vi "Correction SPOT Open.vi"(8 "error in (no error)":errorcluster, 11 "VISA resource name":refnum<visa-resource-name>) -> (0 "error out":errorcluster, 3 "VISA resource name out":refnum<visa-resource-name>)   [LabVIEW 2014, in "LCR Meter.lvlib"]
doc: "Executes the OPEN correction data measure for the specified frequency correction."
uses:
  <instrlib>/LCR Meter/Examples/LCR Meter Acquire Single_1 Folder/LCR Meter.lvlib
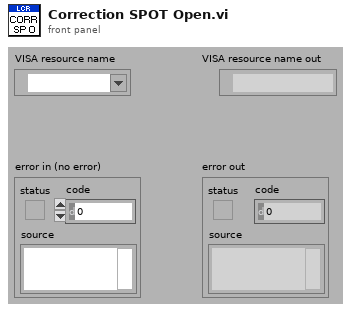
[diagram p1: front panel]
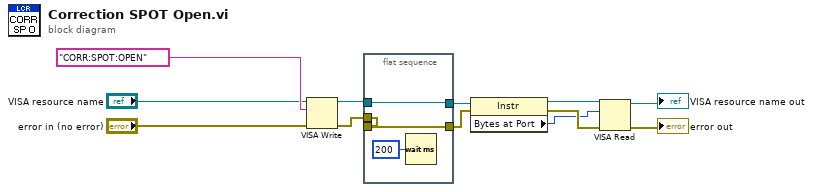
[diagram p0: block diagram]
diagram:
  n1 = VISA Write(VISA resource name="VISA resource name", write buffer="CORR:SPOT:OPEN", error in (no error)="error in (no error)") -> (VISA resource name out=w4:refnum<visa-resource-name>, error out=w3:errorcluster)  [unwired: 1 out]
  n2 = flat-sequence {
    tunnel: w4 -> [w15]
    tunnel: [w13] -> _
    tunnel: [w15] -> w9
    tunnel: [w13] -> w8
    tunnel: w3 -> [w13]
    frame #0 {
      n3 = Wait (ms)(milliseconds to wait=u32 200) -> ()  [unwired: 1 out]
    }
  }
  n4 = property class="Instr"(reference=w9, error in=w8) -> (reference out=w7:refnum<visa-resource-name>, error out=w6:errorcluster, "Bytes at Port"=w5:u32)
  n5 = VISA Read(VISA resource name=w7, byte count=w5, error in (no error)=w6) -> (VISA resource name out=→"VISA resource name out":refnum<visa-resource-name>, error out=→"error out":errorcluster)  [unwired: 2 out]
